vi "L1_LinearThresholdScan.vi"(0 "VISA In":refnum<visa-resource-name>="AgilentOsciloscope", 1 "Adder Register":i32=99, 2 "Vin":dbl=0.1, 3 "File path In":path=path "C:/Users/omartinez/Desktop/L0nL1_Results/L1_SN_00353_DT_Adder_Test.csv", 5 "ID In":refnum<k5>, 7 "Error In":errorcluster, 9 "Threshold Limits In":i16[](array[numeric])=[0, 512], 11 "Channel/Mode":i32=2, 12 "Adder Test?":bool=TRUE, 13 "Digital Output":i32=1) -> (4 "ID out":refnum<k5>, 6 "VISA Out":refnum<visa-resource-name>="AgilentOsciloscope", 10 "Threshold \nLimits Out":i16[](array[numeric])=[66, 67], 15 "Error Out":errorcluster)   [LabVIEW 2012]
uses:
  Sum_Abrilader/L0_Sum_Adder Folder/C/Program Files/National Instruments/LabVIEW 2012/instr.lib/Agilent 8000 Series/Public/Data/Low Level/Fetch Measurement (More).vi
  <vilib>/Utility/file.llb/Write To Spreadsheet File (DBL).vi
  <instrlib>/Agilent 8000 Series/Agilent 8000 Series.lvlib
panel:
  out "DAC Value":i32
  out "Current Threshold \nLimits Out":i16[](array[numeric])=[66, 67]
  out "Waveform Chart":dbl[](graph)
  out "IPR_count 2":u32
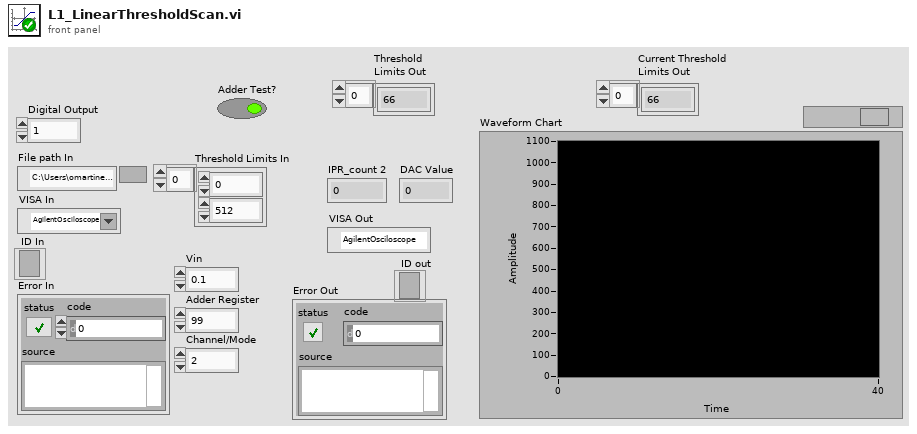
[diagram p1: front panel]
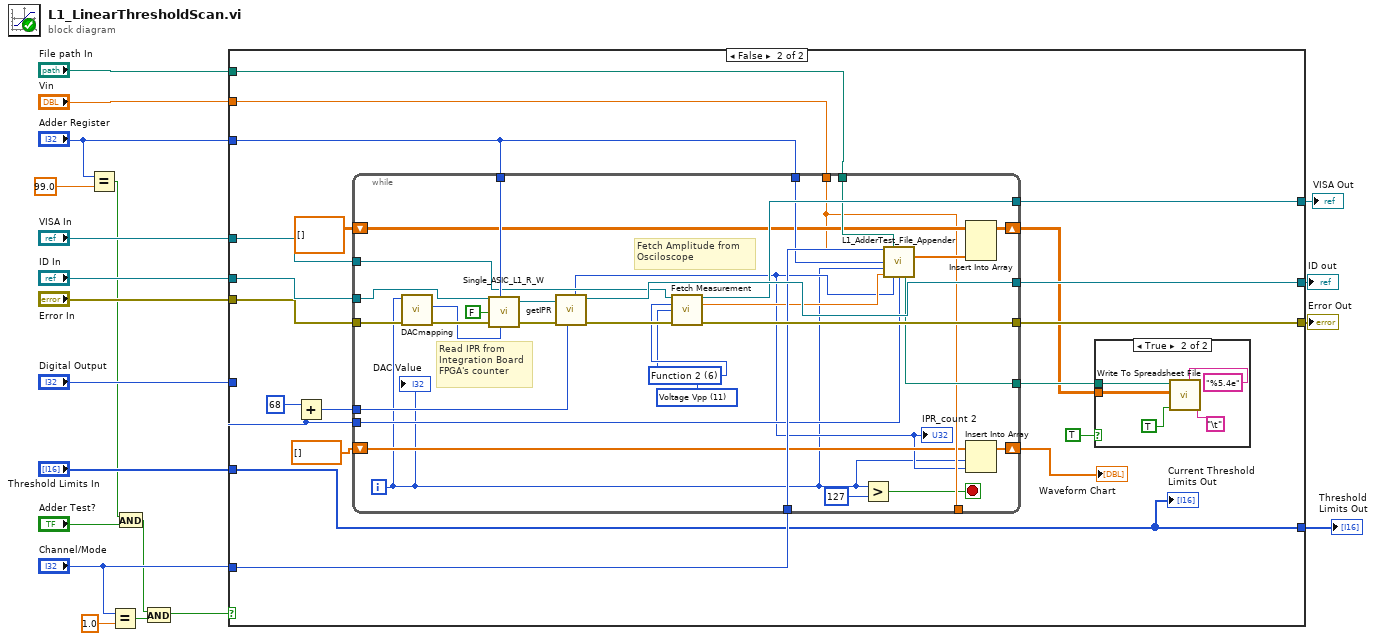
[diagram p0: block diagram]
diagram:
  n1 = Equal?(x="Adder Register", y=99.0) -> (x = y?=w2:bool)
  n2 = Equal?(x="Channel/Mode", y=1.0) -> (x = y?=w8:bool)
  n3 = And(x=w2, y="Adder Test?") -> (x .and. y?=w1:bool)
  n4 = And(x=w1, y=w8) -> (x .and. y?=w9:bool)
  n5 = case shown="False" w9 {
    tunnel: "VISA In" -> [w24 w33]
    tunnel: "ID In" -> [w23 w32]
    tunnel: "Error In" -> [w22 w27]
    tunnel: "Threshold Limits In" -> [w21 w31]
    tunnel: "Digital Output" -> [_ w30]
    tunnel: [w22 w44] -> w15
    tunnel: "Vin" -> [_ w43]
    tunnel: "File path In" -> [_ w42]
    tunnel: [w23 w41] -> w12
    tunnel: "Adder Register" -> [_ w40]
    tunnel: [w21 w31] -> w11
    tunnel: "Channel/Mode" -> [_ w39]
    tunnel: [w24 w38] -> w10
    frame True {
    }
    frame False {
      n6 = Add(x=68, y=w30) -> (x+y=w29:i32)
      n7 = while {
        tunnel: w27 -> [w71]
        tunnel: w32 -> [w70]
        tunnel: w29 -> [w69]
        tunnel: [w67] -> w44
        tunnel: w43 -> [w53]
        tunnel: w42 -> [w62]
        tunnel: w40 -> [w60]
        tunnel: [w66] -> w41
        tunnel: w40 -> [w65]
        tunnel: w33 -> [w64]
        tunnel: w39 -> [w61]
        tunnel: [w63] -> w38
        tunnel: w30 -> [w58]
        tunnel: [w57] -> w37
        shift-right: [w55] -> w36
        shift-left: dbl[][] [] -> [w54]
        tunnel: [w53] -> _
        shift-right: [w52] -> w35
        shift-left: dbl[] [] -> [w51]
        i -> [w47]
        stop <- w49 stop-if-true
        w45 = 11 items=["Rise Time", "Fall Time", "Frequency", "Period", "Voltage RMS(AC)", "Voltage RMS(DC)", "Voltage RMS (AC,cycle)", "Voltage RMS (DC,cycle)", "Voltage Max", "Voltage Min", "Voltage Middle", "Voltage Vpp", "Voltage High", "Voltage Low", "Voltage Average", "Voltage Average (cycle)", "Width Negative", "Width Positive", "Duty Cycle Positive", "Amplitude", "Overshoot", "Preshoot", "Voltage Base", "Voltage Upper", "Time Max", "Time Min", "Color Grade Crossing", "Color Grade Eye Width", "Color Grade Eye Height", "Color Grade Eye Q-Factory", "Color Grade Eye Duty Cycle Distortion(Percent)", "Color Grade Eye Duty Cycle Distortion(Time)", "Color Grade Eye Jitter(PP)", "Color Grade Eye Width(RMS)", "Cycle-cycle Duty Jitter(Rising)", "Cycle-cycle Duty Jitter(Falling)", "Cycle-cycle Jitter(Rising)", "Cycle-cycle Jitter(Falling)", "Cycle-cycle - Width", "Cycle-cycle + Width", "Date Rate", "Unit Interval", "FFT Delta Frequency", "FFT Delta Magnitude", "FFT Frequency", "FFT Magnitude", "Slew Rate", "Area (Entire Display)", "Area(Single Cycle)", "Duty Cycle (Rising)", "Duty Cycle (Falling)"] ("Measurement Function (0: Rise Time)")
        w46 = 6 items=["Channel 1"=1, "Channel 2"=2, "Channel 3"=3, "Channel 4"=4, "Function 1"=5, "Function 2"=6, "Function 3"=7, "Function 4"=8, "Memory 1"=9, "Memory 2"=10, "Memory 3"=11, "Memory 4"=12] ("Channel (1: Channel 1)")
        # "Fetch Amplitude from\nOsciloscope"
        # "Read IPR from \nIntegration Board\nFPGA's counter"
        n8 = call "DACmapping.vi"("error in (no error)"=w71, "DAC_TH"=w47) -> ("error out"=w75:errorcluster, "COMB DEC"=w74:u32)  [unwired: 8 in]
        n9 = call "Single_ASIC_L1_R_W.vi"("connection ID"=w70, "Register or channel"=w65, "RD/#WR"=FALSE, "error in (no error)"=w75, "Data"=w74) -> ("connection ID out"=w72:refnum<k5>, "error out"=w73:errorcluster)  [unwired: 1 in, 2 out]
        n10 = call "getIPR.vi"("Address"=w69, "error in"=w73, "connection ID"=w72) -> ("error out"=w68:errorcluster, "connection ID out"=w66:refnum<k5>, "IPR_count"=w50:u32)  [unwired: 5 in, 1 out]
        "IPR_count 2" <- w50
        n11 = call-poly "Fetch Measurement.vi"("VISA resource name"=w64, "Channel (1: Channel 1)"=w46, "Measurement Function (0: Rise Time)"=w45, "error in (no error)"=w68) -> ("VISA resource name out"=w63:refnum<visa-resource-name>, "Measurement"=w59:dbl, "error out"=w67:errorcluster)  [unwired: 9 in]
        n12 = Greater?(x=w47, y=i16 127) -> (0:w49:bool)
        n13 = call "L1_AdderTest_File_Appender.vi"("Vin"=w53, "file path (dialog if empty)"=w62, "CH"=w61, "Active Adder"=w60, "DAC Level"=w47, "Vmeas"=w59, "IPR"=w50, "Digital Output"=w58) -> ("appended array"=w56:dbl[], "file path (dialog if empty) 2"=w57:path)  [unwired: 6 in]
        n14 = Insert Into Array(array=w54, new element=w56) -> (w55:dbl[][])  [unwired: 2 in]
        n15 = Insert Into Array(array=w51, index=w47, new element=w50) -> (w52:dbl[])
        "DAC Value" <- w47
      }
      "Waveform Chart" <- w35
      n16 = case shown="True" TRUE {
        tunnel: w37 -> [_ w80]
        tunnel: w36 -> [_ w79]
        frame False {
        }
        frame True {
          n17 = call-poly <vilib>:"Write To Spreadsheet File.vi"("delimiter (\\t)"="\t", "format (%.;%.3f)"="%5.4e" ("format (%.3f)"), "append to file? (new file:F)"=TRUE, "2D data"=w79, "file path (dialog if empty)"=w80) -> ()  [unwired: 3 in, 1 out]
        }
      }
      "Current Threshold \nLimits Out" <- w31
    }
  }
  "Threshold \nLimits Out" <- w11
  "Error Out" <- w15
  "ID out" <- w12
  "VISA Out" <- w10
